vi "Recieve Calibration.vi"(8 "error in (no error)":errorcluster, 11 "RP Communicator in":refnum<class "RP Communicator.lvclass">) -> (0 "error out":errorcluster, 2 "Calibration":T1 {"magic" format="%x"}, 3 "RP Communicator out":refnum<class "RP Communicator.lvclass">)   [LabVIEW 2019, in "RP Communicator.lvclass"]
uses:
  RP Communicator.lvclass
  RP EEPROM Calibration.ctl
  RP Command.ctl
  RP Communicator.lvclass/RP Communicator.ctl
  Write RP EEPROM Calibration.vi
  Read RP EEPROM Calibration.vi
  Read Timeout.vi
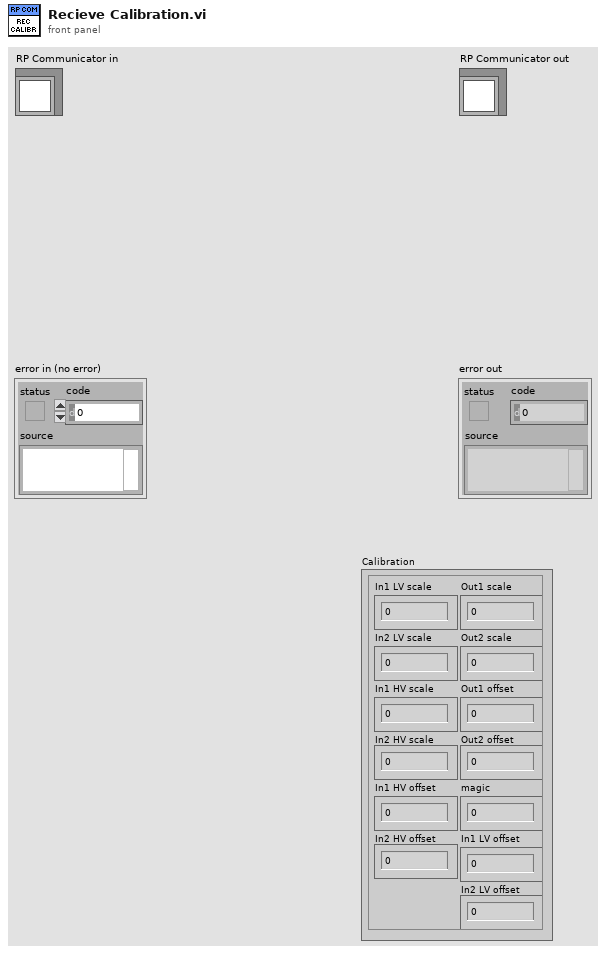
[diagram p1: front panel]
types:
  T1 = typedef "RP EEPROM Calibration.ctl" = cluster{"In1 LV scale":u32, "In2 LV scale":u32, "In1 HV scale":u32, "In2 HV scale":u32, "In1 HV offset":i32, "In2 HV offset":i32, "Out1 scale":u32, "Out2 scale":u32, "Out1 offset":i32, "Out2 offset":i32, "magic":u32, "In1 LV offset":i32, "In2 LV offset":i32}
  T2 = typedef "RP Command.ctl" = enum16{"Reset", "Read IDN", "Stop server", "Get status", "Get temperature", "Connect client", "Arm", "Software trigger", "Get whole buffer", "Get chunk", "System call", "Get config", "Set config", "Recieve data", "Recieve Calibartion", "Transmit data"}
  T3 = enum16{"big-endian, network order", "native, host order", "little-endian"}
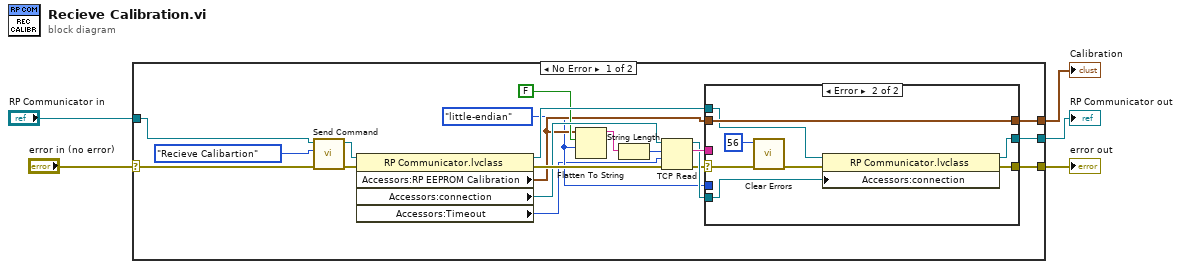
[diagram p0: block diagram]
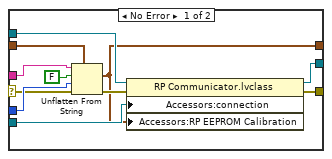
[diagram p2: hidden frame]
diagram:
  n1 = case shown="No Error" "error in (no error)" {
    selector: "error in (no error)" -> [w18 w46]
    tunnel: [w17 w46] -> w4
    tunnel: [w15 w45] -> w2
    tunnel: "RP Communicator in" -> [w16 w45]
    tunnel: [w14 _] -> w1
    frame No Error {
      w9 = T3."little-endian" ("byte order (0:big-endian, network order)")
      n2 = call-dynamic "Send Command.vi"("error in (no error)"=w18, "Command number"=RP_Command."Recieve Calibartion", "RP Communicator in"=w16) -> ("error out"=w23:errorcluster, "RP Communicator out"=w13:refnum<class "RP Communicator.lvclass">)  [unwired: 7 in]
      n3 = property class="RP Communicator.lvclass"(reference=w13, error in=w23) -> (reference out=w25:refnum<class "RP Communicator.lvclass">, error out=w21:errorcluster, "Accessors:RP EEPROM Calibration"=w10:T1, "Accessors:connection"=w19:refnum<k5>, "Accessors:Timeout"=w7:i32)
      n4 = Flatten To String(anything=w10, prepend array or string size? (T)=FALSE, byte order (0:big-endian, network order)=w9) -> (data string=w11:string)  [unwired: 1 in, 2 out]
      n5 = String Length(string=w11) -> (length=w8:i32)
      n6 = TCP Read(connection ID=w19, bytes to read=w8, error in (no error)=w21, 9:w7) -> (connection ID out=w20:refnum<k5>, data out=w24:string, error out=w6:errorcluster)  [unwired: 1 in]
      n7 = case shown="Error" w6 {
        selector: w6 -> [w26 w44]
        tunnel: w25 -> [w36 w39]
        tunnel: w24 -> [w34 _]
        tunnel: w20 -> [w33 w37]
        tunnel: [w31 w40] -> w17
        tunnel: [w30 w38] -> w15
        tunnel: [w29 w43] -> w14
        tunnel: w10 -> [w28 w43]
        tunnel: w9 -> [w27 _]
        frame No Error {
          n8 = Unflatten From String(type=w28, binary string=w34, data includes array or string size? (T)=FALSE, byte order (0:big-endian, network order)=w27, error in (no error)=w26) -> (value=w29:T1, error out=w32:errorcluster)  [unwired: 1 out]
          n9 = property class="RP Communicator.lvclass"(reference=w36, error in=w32, "Accessors:connection"=w33, "Accessors:RP EEPROM Calibration"=w29) -> (reference out=w30:refnum<class "RP Communicator.lvclass">, error out=w31:errorcluster)
        }
        frame Error {
          n10 = call <vilib>:"Clear Errors.vi"("error in (no error)"=w44, "specific error code to clear (0: all)"=56) -> ("error out"=w42:errorcluster)  [unwired: 4 in, 1 out]
          n11 = property class="RP Communicator.lvclass"(reference=w39, error in=w42, "Accessors:connection"=w37) -> (reference out=w38:refnum<class "RP Communicator.lvclass">, error out=w40:errorcluster)
        }
      }
    }
    frame Error {
    }
  }
  "error out" <- w4
  "RP Communicator out" <- w2
  "Calibration" <- w1
